vi "Read RT FIFO.vi"   [LabVIEW 2017, in "Data Sharing Framework Engine.lvlib" / "Engine Interface.lvclass"]
uses:
  Engine Interface.lvclass
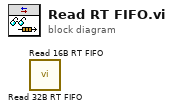
[diagram p0: block diagram]
diagram:
  n1 = call "Read 32B RT FIFO.vi"() -> ()  [unwired: 7 in, 5 out]
  n2 = call "Read 16B RT FIFO.vi"() -> ()  [unwired: 7 in, 5 out]
